vi "Launch Analog Reader.vi"(8 "error in (no error)":errorcluster, 11 "Root Tester in":refnum<class "Root Tester.lvclass">) -> (0 "error out":errorcluster, 3 "Root Tester out":refnum<class "Root Tester.lvclass">)   [LabVIEW 2024, in "Root Tester.lvlib" / "Root Tester.lvclass"]
uses:
  Root Tester.lvclass
  C:/Program Files (x86)/National Instruments/LabVIEW 2024/vi.lib/ActorFramework/Actor/Actor.lvclass
  DAQmx Actor/Analog Reader/Analog Reader.lvclass
  Root Tester.lvclass/Root Tester.ctl
  <vilib>/DAQmx/create/channels.llb/DAQmx Create Channel (AI-Voltage-Basic).vi
  <vilib>/DAQmx/configure/timing.llb/DAQmx Timing (Sample Clock).vi
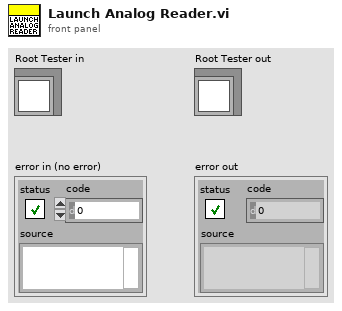
[diagram p1: front panel]
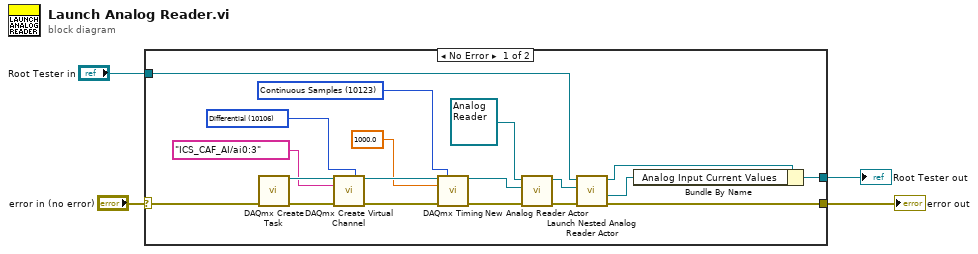
[diagram p0: block diagram]
diagram:
  n1 = case shown="No Error" "error in (no error)" {
    selector: "error in (no error)" -> [w18 w25]
    tunnel: [w15 w25] -> w3
    tunnel: [w6 w24] -> w1
    tunnel: "Root Tester in" -> [w23 w24]
    frame No Error {
      w8 = 10123 items=["Finite Samples"=10178, "Continuous Samples"=10123, "Hardware Timed Single Point"=12522] ("sample mode")
      w13 = 10106 items=["Default"=-1, "RSE"=10083, "NRSE"=10078, "Differential"=10106, "Pseudodifferential"=12529] ("input terminal configuration")
      n2 = call <vilib>:"DAQmx Create Task.vi"("error in"=w18) -> ("task out"=w22:refnum<k21>, "error out"=w19:errorcluster)  [unwired: 13 in]
      n3 = call-poly <vilib>:"DAQmx Create Virtual Channel.vi"("task in"=w22, "input terminal configuration"=w13, "physical channels"=tag "ICS_CAF_AI/ai0:3", "error in"=w19) -> ("task out"=w14:refnum<k21>, "error out"=w10:errorcluster)  [unwired: 10 in]
      n4 = call-poly <vilib>:"DAQmx Timing.vi"("task/channels in"=w14, "sample mode"=w8, "rate"=1000.0, "error in"=w10) -> ("task out"=w12:refnum<k21>, "error out"=w11:errorcluster)  [unwired: 10 in]
      n5 = call-dynamic "New Analog Reader Actor.vi"("error in (no error)"=w11, "DAQmx Task"=w12, "Analog Reader in"=refnum<class "Analog Reader.lvclass"> refnum) -> ("error out"=w16:errorcluster, "Analog Reader out"=w17:refnum<class "Analog Reader.lvclass">)  [unwired: 7 in]
      n6 = call "Launch Nested Analog Reader Actor.vi"("error in (no error)"=w16, "Nested Analog Reader Actor"=w17, "Caller Actor in"=w23) -> ("error out"=w15:errorcluster, "High Speed Data Queue"=w5:refnum<queue>, "Caller Actor out"=w7:refnum<class "Root Tester.lvclass">)  [unwired: 5 in, 1 out]
      n7 = Bundle By Name(cluster=w7, "Analog Input Current Values"=w5) -> (w6:refnum<class "Root Tester.lvclass">)
    }
    frame Error {
    }
  }
  "error out" <- w3
  "Root Tester out" <- w1
